vi "Sliding Menu Initialize.vi"(3 "Container State":T6, 4 "Previous State":variant, 5 "Previous Version":T5) -> (2 "Current State":T1={"Numeric"=0.0, "Array of Button References"=[], "Space Between Menu Buttons"=0, "Number of Menu Buttons"=0, "Array of Button Names"=[], "Most Recent Vertical Position"=0, "This VI"=refnum, "Current Action"=enum."Not Moving", "Most Recent Distance Traveled"=0, "Method"=enum."Move Up", "Data In"=0})   [LabVIEW 2011, in "Sliding Menu Library.lvlib" / "Sliding Menu XControl.xctl"]
uses:
  Sliding Menu XControl.xctl
  Sliding Menu State.ctl
  Menu Button Library/Menu Button xControl/Menu Button xControl.xctl
  Sliding Menu SubVIs/Sliding Menu Type Definitions/Current User Action.ctl
  Sliding Menu Methods.ctl
  Sliding Menu Data.ctl
  <vilib>/_xctls/Container State.ctl
  <vilib>/_xctls/Version.ctl
  <vilib>/_xctls/XControlSupport.lvlib
  Sliding Menu Library.lvlib
panel:
  in  "Default Indicator State":T1={"Numeric"=0.0, "Array of Button References"=[], "Space Between Menu Buttons"=0, "Number of Menu Buttons"=0, "Array of Button Names"=[], "Most Recent Vertical Position"=0, "This VI"=refnum, "Current Action"=enum."Not Moving", "Most Recent Distance Traveled"=0, "Method"=enum."Move Up", "Data In"=0}
  in  "Default Control State":T1={"Numeric"=0.0, "Array of Button References"=[], "Space Between Menu Buttons"=0, "Number of Menu Buttons"=0, "Array of Button Names"=[], "Most Recent Vertical Position"=0, "This VI"=refnum, "Current Action"=enum."Not Moving", "Most Recent Distance Traveled"=0, "Method"=enum."Move Up", "Data In"=0}
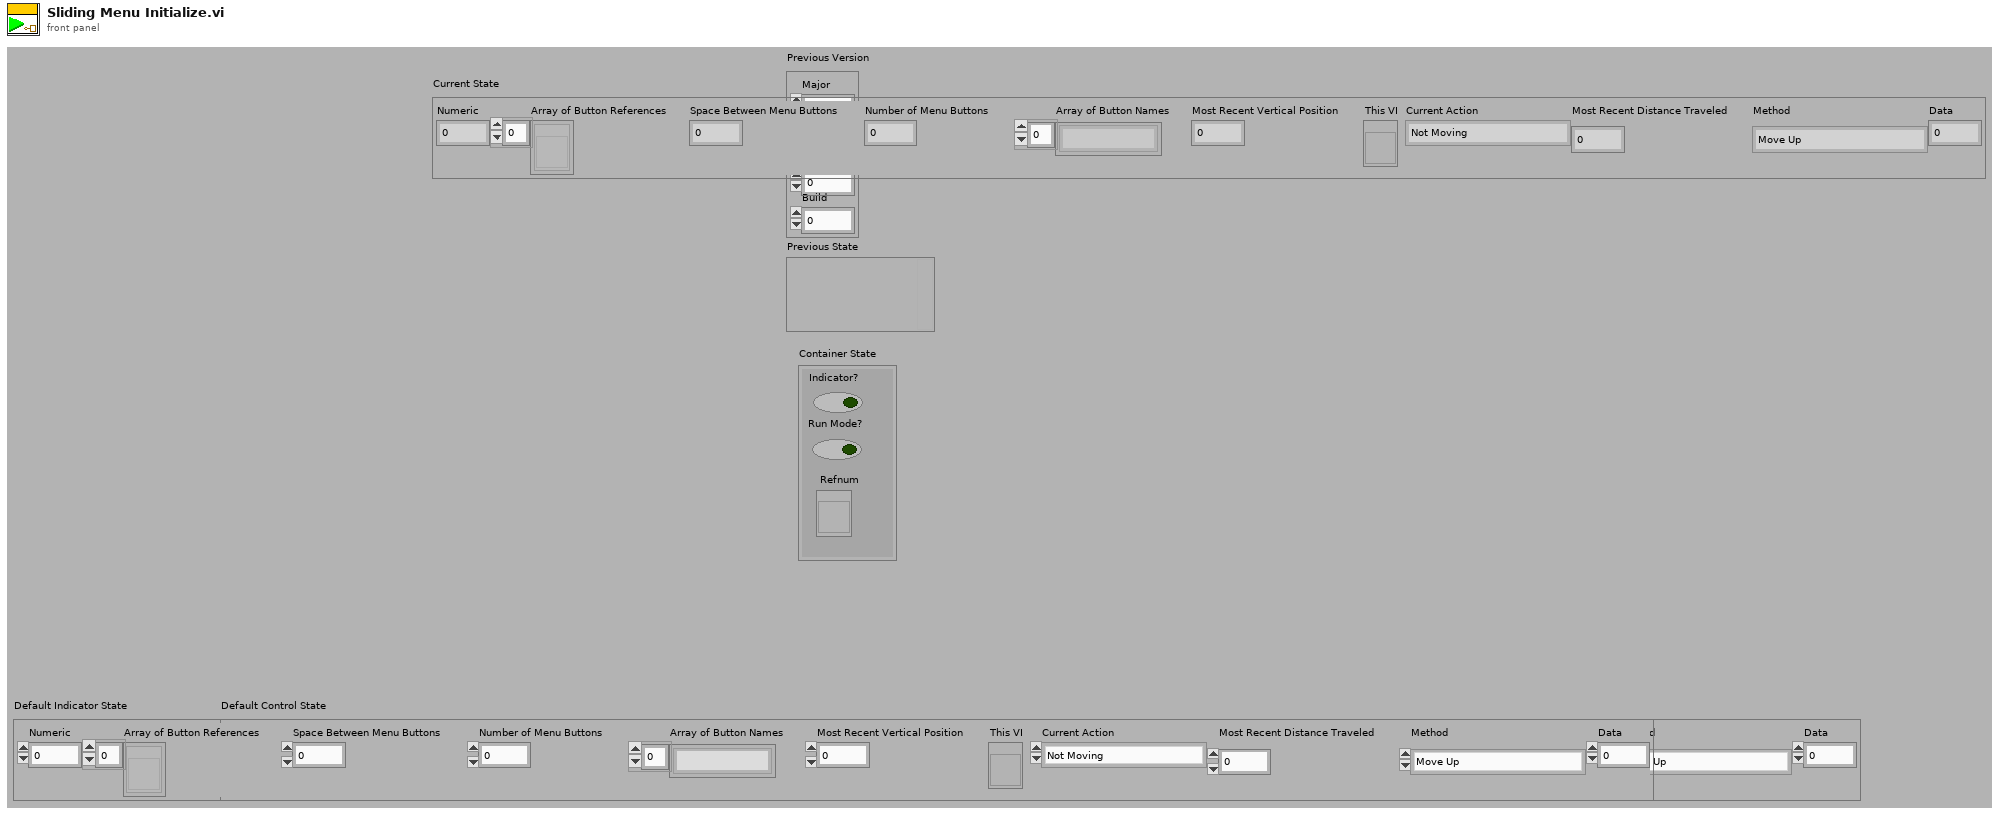
[diagram p1: front panel]
types:
  T1 = typedef "Sliding Menu Library.lvlib/Sliding Menu XControl.xctl/Sliding Menu State.ctl" = cluster{"Numeric":dbl, "Array of Button References":refnum<vi>[], "Space Between Menu Buttons":i32, "Number of Menu Buttons":i32, "Array of Button Names":string[], "Most Recent Vertical Position":i32, "This VI":refnum<vi>, "Current Action":T2, "Most Recent Distance Traveled":i32, "Method":T3, "Data In":T4}
  T2 = typedef "Sliding Menu Library.lvlib/Current User Action.ctl" = enum16{"Not Moving", "Mouse Down", "Mouse Up No Dragging", "Bounce Up Needed", "Bounce Down Needed", "Dragging", "Easing"}
  T3 = typedef "Sliding Menu Methods.ctl" = enum16{"Resize", "Move Up", "Move Down", "Move to 0"}
  T4 = typedef "Sliding Menu Library.lvlib/Sliding Menu XControl.xctl/Sliding Menu Data.ctl" = i32
  T5 = typedef "XControlSupport.lvlib/Version.ctl" = cluster{"Major":u16, "Minor":u16, "Fix":u16, "Build":u16}
  T6 = typedef "XControlSupport.lvlib/Container State.ctl" = cluster{"Indicator?":bool, "Run Mode?":bool, " Refnum":refnum<vi>}
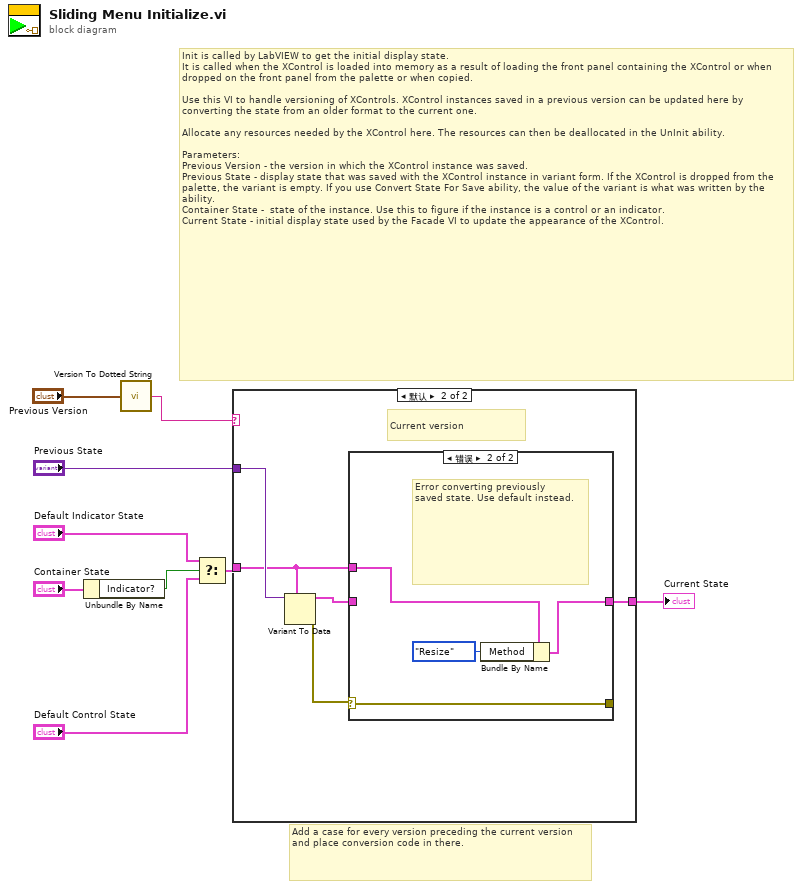
[diagram p0: block diagram]
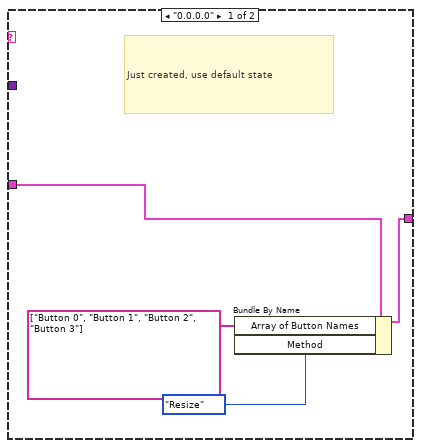
[diagram p2: hidden frame]
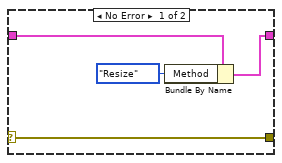
[diagram p3: hidden frame]
diagram:
  # "Add a case for every version preceding the current version and place conversion code in there."
  # "Init is called by LabVIEW to get the initial display state.\nIt is called when the XControl is loaded into memory as a result of loading the front panel containing the XControl or when dropped on the front panel from the palette or when copied.\n\nUse this VI to handle versioning of XControls. XControl instances saved in a previous version can be updated here by converting the state from an older format to the current one.\n\nAllocate any resources needed by the XControl here. The resources can then be deallocated in the UnInit ability.\n\nParameters:\nPrevious Version - the version in which the XControl instance was saved.\nPrevious State - display state that was saved with the XControl instance in variant form. If the XControl is dropped from the palette, the variant is empty. If you use Convert State For Save ability, the value of the variant is what was written by the ability. \nContainer State -  state of the instance. Use this to figure if the instance is a control or an indicator.\nCurrent State - initial display state used by the Facade VI to update the appearance of the XControl."
  n1 = Unbundle By Name("Container State") -> ("Indicator?"=w4:bool)
  n2 = call <vilib>:"Version To Dotted String.vi"("Version"="Previous Version") -> ("String Version"=w1:string)
  n3 = Select(t="Default Indicator State", s=w4, f="Default Control State") -> (s? t:f=w3:T1)
  n4 = case shown="默认" w1 {
    tunnel: "Previous State" -> [_ w18]
    tunnel: [w12 w14] -> w8
    tunnel: w3 -> [w13 w15]
    frame "0.0.0.0" {
      # "Just created, use default state"
      n5 = Bundle By Name(cluster=w13, "Array of Button Names"=string[] ["Button 0", "Button 1", "Button 2", "Button 3"], "Method"=Sliding_Menu_Methods."Resize") -> (w12:T1)
    }
    frame Default {
      # "Current version"
      n6 = Variant To Data(type=w15, Variant=w18) -> (data=w16:T1, error out=w17:errorcluster)  [unwired: 1 in]
      n7 = case shown="错误" w17 {
        selector: w17 -> [w22 w26]
        tunnel: w16 -> [w21 _]
        tunnel: [w20 w23] -> w14
        tunnel: w15 -> [_ w24]
        tunnel: [w22 w26] -> _
        frame No Error {
          n8 = Bundle By Name(cluster=w21, "Method"=Sliding_Menu_Methods."Resize") -> (w20:T1)
        }
        frame Error {
          # "Error converting previously \nsaved state. Use default instead."
          n9 = Bundle By Name(cluster=w24, "Method"=Sliding_Menu_Methods."Resize") -> (w23:T1)
        }
      }
    }
  }
  "Current State" <- w8
